vi "Configure Alternation Trigger.vi"   [LabVIEW 2010, in "Agilent DSO1000 Series.lvlib"]
doc: "Selects the type of alternation trigger."
uses:
  <instrlib>/Agilent DSO1000 Series/Agilent DSO1000 Series.lvlib
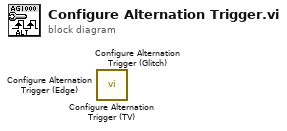
[diagram p0: block diagram]
diagram:
  n1 = call <instrlib>:"Configure Alternation Trigger (TV).vi"() -> ()  [unwired: 14 in, 2 out]
  n2 = call <instrlib>:"Configure Alternation Trigger (Glitch).vi"() -> ()  [unwired: 14 in, 2 out]
  n3 = call <instrlib>:"Configure Alternation Trigger (Edge).vi"() -> ()  [unwired: 14 in, 2 out]
